vi "Configure Serial Watchdog.vi"(8 "error in (no error)":errorcluster, 10 "time, s (0 = disabled)":u16, 11 "Comdel in":refnum<class "PL Comdel CX.lvclass">) -> (0 "error out":errorcluster, 2 "time, s":u16, 3 "Comdel out":refnum<class "PL Comdel CX.lvclass">)   [LabVIEW 2015, in "PL Comdel CX.lvclass"]
doc: "Configures serial watchdog <b>time</b>. If RF power is enabled no RF power enable commands are sent during this time, RF power is disabled. Zero time value disables the watchdog."
uses:
  PL Comdel CX.lvclass
  PL Comdel CX.lvclass/PL Comdel CX.ctl
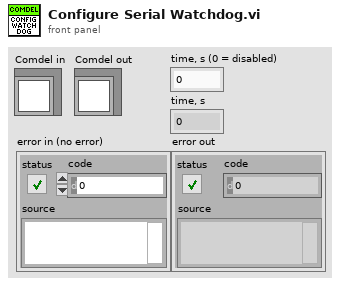
[diagram p1: front panel]
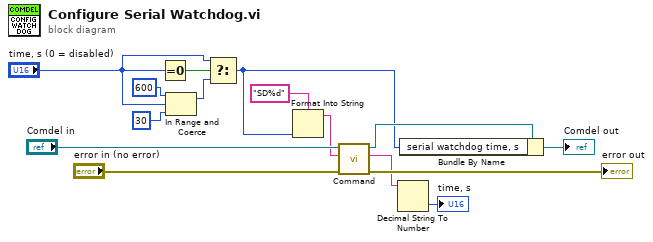
[diagram p0: block diagram]
diagram:
  n1 = Equal To 0?(x="time, s (0 = disabled)") -> (x = 0?=w9:bool)
  n2 = In Range and Coerce(upper limit=u16 600, x="time, s (0 = disabled)", lower limit=u16 30) -> (coerced(x)=w5:u16)  [unwired: 1 out]
  n3 = Select(t="time, s (0 = disabled)", s=w9, f=w5) -> (s? t:f=w3:u16)
  n4 = Format Into String(format string="SD%d", w3) -> (resulting string=w4:string)  [unwired: 2 in, 1 out]
  n5 = call "Command.vi"("error in (no error)"="error in (no error)", "command"=w4, "Comdel in"="Comdel in") -> ("error out"=→"error out":errorcluster, "response data"=w2:string, "Comdel out"=w12:refnum<class "PL Comdel CX.lvclass">)  [unwired: 6 in]
  n6 = Decimal String To Number(string=w2) -> (number=→"time, s":i32)  [unwired: 2 in, 1 out]
  n7 = Bundle By Name(cluster=w12, "serial watchdog time, s"=w3) -> (→"Comdel out":refnum<class "PL Comdel CX.lvclass">)
